vi "Write CSV with Header Demo.vi"() -> ()   [LabVIEW 2020]
panel:
  in  "file path":path
  in  "Boolean":bool
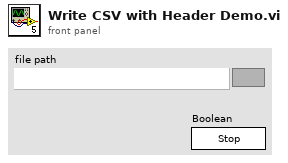
[diagram p1: front panel]
types:
  T1 = enum16{"open", "replace", "create", "open or create", "replace or create", "replace or create with confirmation"}
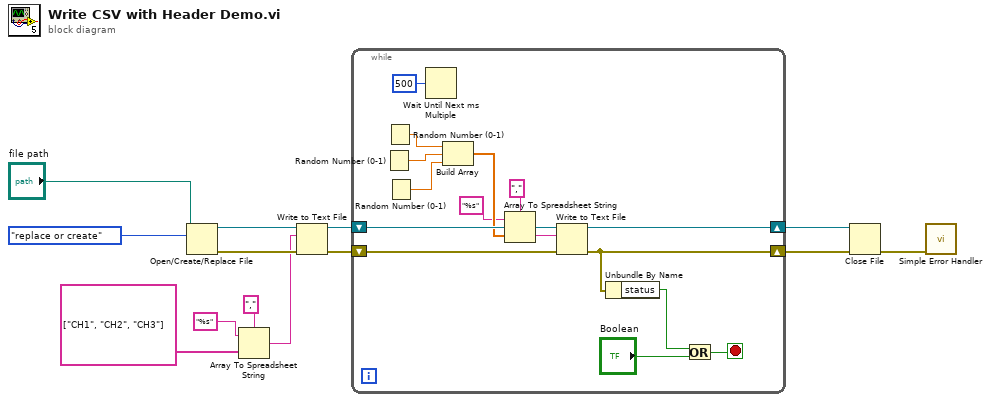
[diagram p0: block diagram]
diagram:
  n1 = Open/Create/Replace File(file path (use dialog)="file path", operation (0:open)=T1."replace or create") -> (refnum out=w8:refnum<file>, error out=w5:errorcluster)  [unwired: 1 in, 4 out]
  n2 = Array To Spreadsheet String(delimiter (Tab)=",", array=string[] ["CH1", "CH2", "CH3"], 3:"%s" ("format string")) -> (spreadsheet string=w1:string)
  n3 = Write to Text File(file (use dialog)=w8, text=w1, error in=w5) -> (refnum out=w7:refnum<file>, error out=w6:errorcluster)  [unwired: 2 out]
  n4 = while {
    shift-right: [w22] -> w12
    shift-left: w6 -> [w24]
    shift-right: [w25] -> w13
    shift-left: w7 -> [w26]
    stop <- w23 stop-if-true
    n5 = Random Number (0-1)() -> (number: 0 to 1=w19:dbl)
    n6 = Random Number (0-1)() -> (number: 0 to 1=w20:dbl)
    n7 = Random Number (0-1)() -> (number: 0 to 1=w18:dbl)
    n8 = Wait Until Next ms Multiple(millisecond multiple=u32 500) -> ()  [unwired: 1 out]
    n9 = Build Array(w20, w19, w18) -> (w17:dbl[])
    n10 = Array To Spreadsheet String(delimiter (Tab)=",", array=w17, 3:"%s" ("format string")) -> (spreadsheet string=w16:string)
    n11 = Write to Text File(file (use dialog)=w26, text=w16, error in=w24) -> (refnum out=w25:refnum<file>, error out=w22:errorcluster)  [unwired: 2 out]
    n12 = Unbundle By Name(w22) -> ("status"=w21:bool)
    n13 = Or(x=w21, y="Boolean") -> (x .or. y?=w23:bool)
  }
  n14 = Close File(refnum=w13, error in=w12) -> (error out=w11:errorcluster)  [unwired: 1 out]
  n15 = call <vilib>:"Simple Error Handler.vi"("error in (no error)"=w11) -> ()  [unwired: 1 in, 8 out]
